vi "Get Build Specification Names.vi"(8 "error in (no error)":errorcluster, 9 "Build specification regexp filter (.*)":string=".*", 10 "Target Name":string, 11 "Project Path":path) -> (0 "error out":errorcluster, 1 "Build specification names with version string":string[](array[string]), 2 "Build spec vections":T1[](array[typedef]), 3 "Build specification names":string[](array[string]), 4 "Build spec references":refnum<vi>[](array[refnum]))   [LabVIEW 2020]
doc: "Obtains build specification names available in project. Can be called only from pre/post builds actions!"
uses:
  <vilib>/AppBuilder/AB_API_Simple/Build Specification Version.ctl
  <vilib>/AppBuilder/AB_API_Simple/Get Build Specification Version (path).vi
  <vilib>/regexp/Match Regular Expression.xnode
  <vilib>/AppBuilder/AB_API_Simple/NI_App_Builder_API.lvlib
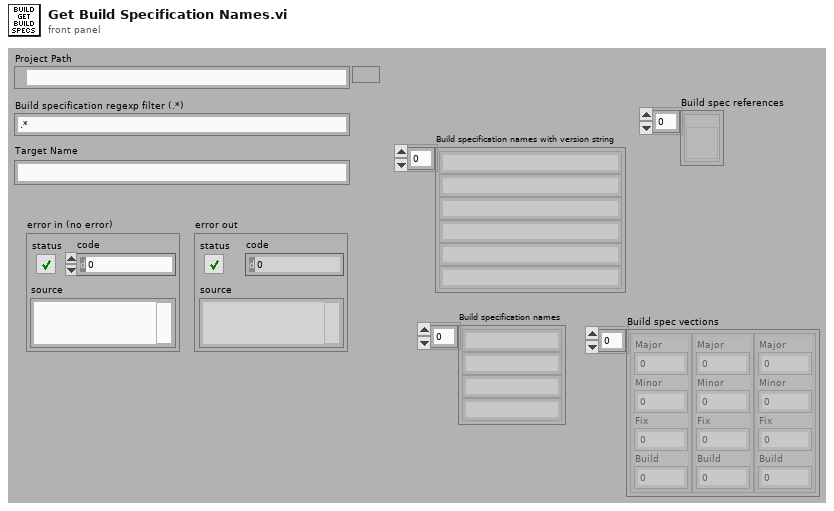
[diagram p1: front panel]
types:
  T1 = typedef "NI_App_Builder_API.lvlib/Build Specification Version.ctl" = cluster{"Major":u16, "Minor":u16, "Fix":u16, "Build":u16}
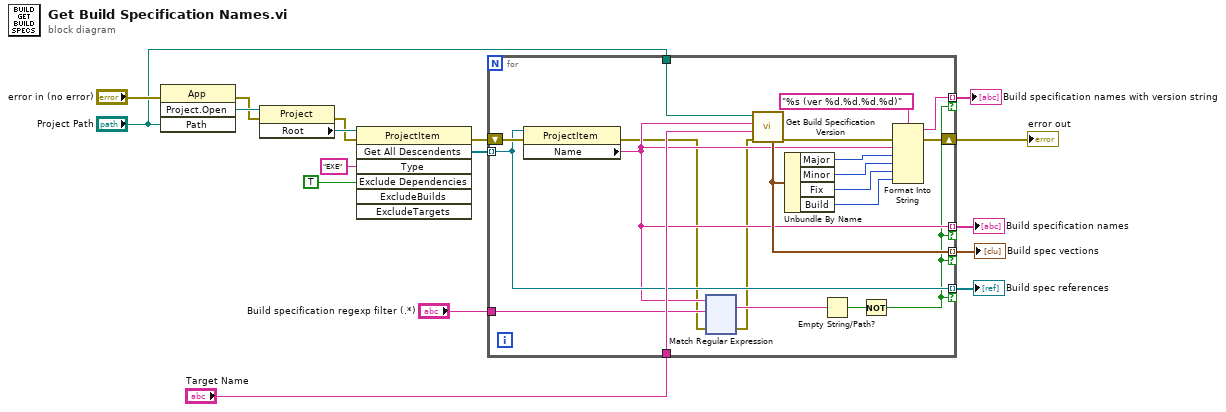
[diagram p0: block diagram]
diagram:
  n1 = invoke class="App" method="Project.Open"(error in="error in (no error)", "Path"="Project Path") -> (error out=w16:errorcluster, "Project:Open"=w17:refnum<vi>)  [unwired: 2 in, 2 out]
  n2 = property class="Project"(reference=w17, error in=w16) -> (error out=w14:errorcluster, "Root"=w15:refnum<vi>)  [unwired: 1 out]
  n3 = invoke class="ProjectItem" method="Get All Descendents"(reference=w15, error in=w14, "Type"="EXE", "Exclude Dependencies"=TRUE ("ExcludeDependencies")) -> (error out=w13:errorcluster, "All Descendents"=w12:refnum<vi>[])  [unwired: 3 in, 5 out]
  n4 = for {
    tunnel: w12 -> [w25] mode=indexing
    tunnel: [w24] -> w4 mode=indexing if=w20
    shift-right: [w33] -> w8
    shift-left: w13 -> [w37]
    tunnel: "Project Path" -> [w36]
    tunnel: "Target Name" -> [w35]
    tunnel: [w27] -> w2 mode=indexing if=w20
    tunnel: [w26] -> w3 mode=indexing if=w20
    tunnel: [w25] -> w1 mode=indexing if=w20
    tunnel: "Build specification regexp filter (.*)" -> [w23]
    n5 = property class="ProjectItem"(reference=w25, error in=w37) -> (error out=w19:errorcluster, "Name"=w24:string)  [unwired: 1 out]
    n6 = xnode "Match Regular Expression"("input string"=w24, "regular expression"=w23, "error in"=w19) -> ("whole match"=w22:string, "error out"=w18:errorcluster)  [unwired: 3 in, 3 out]
    n7 = call-poly <vilib>:"Get Build Specification Version.vi"("error in (no error)"=w18, "Name of target (My Computer)"=w35, "Name of build specification"=w24, "Path to project"=w36) -> ("error out"=w34:errorcluster, "Build Specification Version"=w27:T1)  [unwired: 6 in]
    n8 = Unbundle By Name(w27) -> ("Major"=w31:u16, "Minor"=w30:u16, "Fix"=w29:u16, "Build"=w28:u16)
    n9 = Empty String/Path?(string/path=w22) -> (empty?=w21:bool)
    n10 = Not(x=w21) -> (.not. x?=w20:bool)
    n11 = Format Into String(format string="%s (ver %d.%d.%d.%d)", error in=w34, w24, w31, w30, w29, w28) -> (resulting string=w26:string, error out=w33:errorcluster)  [unwired: 1 in]
  }
  "error out" <- w8
  "Build specification names" <- w4
  "Build specification names with version string" <- w3
  "Build spec vections" <- w2
  "Build spec references" <- w1
